vi "Execute Move Labels.vi"(6 "Mouse Position":T1 caption="鼠标位置", 8 "User VI Ref":refnum<vi> caption="用户VI引用", 9 "Menu Item Tag Suffix":string caption="菜单项标签后缀", 10 "Remaining Items":refnum<vi>[](array[refnum]) caption="剩余项", 11 "Affected Items":T2 caption="受影响的项") -> (0 "Fail transaction?":bool caption="操作失败？")   [LabVIEW 2020]
doc: "该VI属于修改LabVIEW快捷菜单部分。这是用户选择快捷菜单时调用的执行VI。该VI执行选中菜单项的操作。"
uses:
  Move Labels.ctl
  <vilib>/Utility/miscctls.llb/LVPositionTypeDef.ctl
panel:
  # "除“受影响的项”之外，前面板上的其他所有控件都已锁定，以防被意外编辑。修改控件名称或类型，而不是“受影响的项”簇的元素将使VI无法作为菜单插件使用。\n\n请参考每个控件的即时帮助了解其用法。"
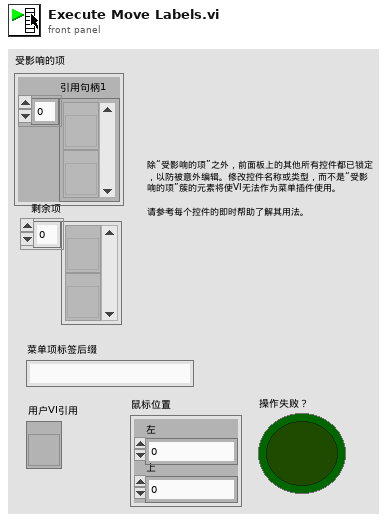
[diagram p1: front panel]
types:
  T1 = typedef "LVPositionTypeDef.ctl" = cluster{"Left":i32, "Top":i32}
  T2 = typedef "Move Labels.ctl" = cluster{"Refnums 1":refnum<vi>[]}
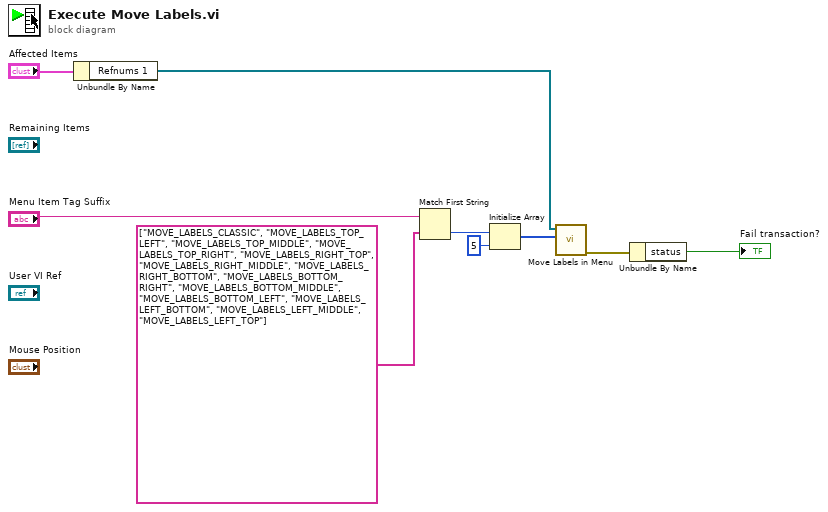
[diagram p0: block diagram]
diagram:
  n1 = Unbundle By Name("Affected Items") -> ("Refnums 1"=w8:refnum<vi>[])
  n2 = Match First String(2:string[] ["MOVE_LABELS_CLASSIC", "MOVE_LABELS_TOP_LEFT", "MOVE_LABELS_TOP_MIDDLE", "MOVE_LABELS_TOP_RIGHT", "MOVE_LABELS_RIGHT_TOP", "MOVE_LABELS_RIGHT_MIDDLE", "MOVE_LABELS_RIGHT_BOTTOM", "MOVE_LABELS_BOTTOM_RIGHT", "MOVE_LABELS_BOTTOM_MIDDLE", "MOVE_LABELS_BOTTOM_LEFT", "MOVE_LABELS_LEFT_BOTTOM", "MOVE_LABELS_LEFT_MIDDLE", "MOVE_LABELS_LEFT_TOP"] ("数组"), 3:"Menu Item Tag Suffix") -> (0:w3:i32)  [unwired: 1 out]
  n3 = Initialize Array(w3, 5 ("维数大小")) -> (w2:i32[])
  n4 = call "Move Labels in Menu.vi"("标签位置"=w2, "图形对象"=w8) -> ("error out"=w7:errorcluster)  [unwired: 9 in]
  n5 = Unbundle By Name(w7) -> ("status"=→"Fail transaction?":bool)
